vi "Get Digital Data.vi"(0 "Input Array":u8[](array[numeric]), 5 "Analog Input":dbl, 7 "Resolution":dbl, 9 "Range":dbl, 11 "Error In":errorcluster) -> (4 "Output Array":u8[](array[numeric]), 15 "Error Out":errorcluster)   [LabVIEW 2021]
doc: "This VI gets the neccessary inputs and gives the digital data out using the formula and gives out as an U8 array."
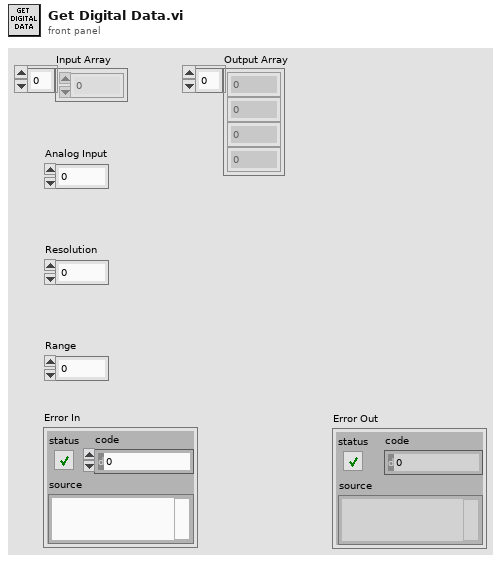
[diagram p1: front panel]
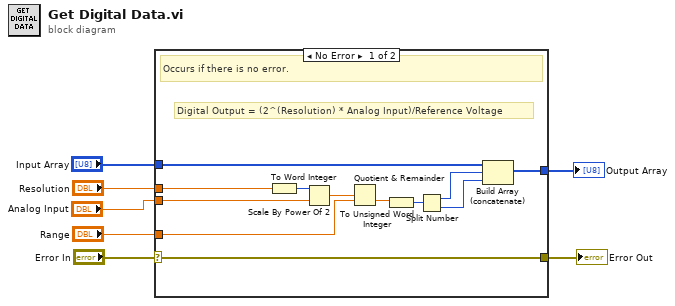
[diagram p0: block diagram]
diagram:
  n1 = case shown="No Error" "Error In" {
    selector: "Error In" -> [w8 w21]
    tunnel: "Input Array" -> [w13 w20]
    tunnel: "Resolution" -> [w12 _]
    tunnel: "Analog Input" -> [w11 _]
    tunnel: "Range" -> [w10 _]
    tunnel: [w9 w20] -> w2
    tunnel: [w8 w21] -> w1
    frame No Error {
      # "Digital Output = (2^(Resolution) * Analog Input)/Reference Voltage"
      # "Occurs if there is no error."
      n2 = To Word Integer(number=w12) -> (16bit integer=w18:i16)
      n3 = Scale By Power Of 2(n=w18, x=w11) -> (x*2^n=w19:dbl)
      n4 = Quotient & Remainder(x=w19, y=w10) -> (floor(x/y)=w17:dbl)  [unwired: 1 out]
      n5 = To Unsigned Word Integer(number=w17) -> (unsigned 16bit integer=w16:u16)
      n6 = Split Number(x=w16) -> (hi(x)=w14:u8, lo(x)=w15:u8)
      n7 = Build Array (concatenate)(w13, w14, w15) -> (w9:u8[])
    }
    frame Error {
      # "Occurs if there is any error."
    }
  }
  "Error Out" <- w1
  "Output Array" <- w2
